vi "OAT Spectral Map.vi"   [LabVIEW 2017, in "SoundVib_OrderTracking.lvlib"]
doc: "Computes a spectral map of the <B>scaled signal [EU]</B> as a function of time or rotational speed. This VI can return the spectral map as a 2D numeric array, a colormap, or a waterfall graph. Wire data to the <B>scaled signal [EU]</B> input to determine the polymorphic instance to use or manually select the instance."
uses:
  <vilib>/addons/Sound and Vibration/Order Analysis/Resample Order Tracking/SoundVib_OrderTracking.lvlib
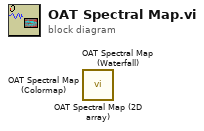
[diagram p0: block diagram]
diagram:
  n1 = call <vilib>:"OAT Spectral Map (2D array).vi"() -> ()  [unwired: 11 in, 5 out]
  n2 = call <vilib>:"OAT Spectral Map (Waterfall).vi"() -> ()  [unwired: 11 in, 5 out]
  n3 = call <vilib>:"OAT Spectral Map (Colormap).vi"() -> ()  [unwired: 11 in, 5 out]
